vi "Any.vi"(8 "input valid":bool=TRUE, 10 "Value":bool, 11 "Reset":bool) -> (0 "output valid":bool, 2 "Any?":bool)   [LabVIEW 2013]
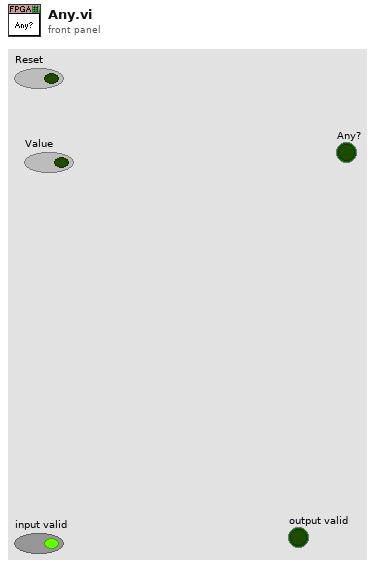
[diagram p1: front panel]
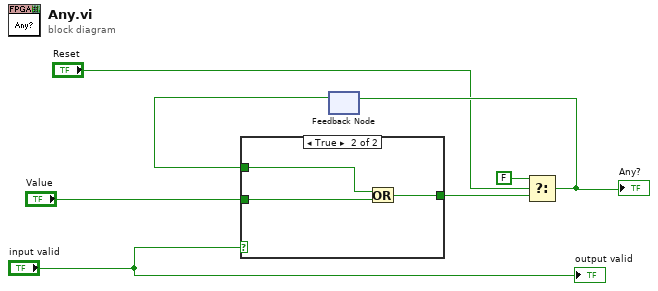
[diagram p0: block diagram]
diagram:
  n1 = feedback #1() -> (w6:bool)  [unwired: 1 in]
  n2 = case shown="True" "input valid" {
    tunnel: "Value" -> [_ w11]
    tunnel: [w8 w10] -> w4
    tunnel: w6 -> [w8 w9]
    frame False {
    }
    frame True {
      n3 = Or(x=w9, y=w11) -> (x .or. y?=w10:bool)
    }
  }
  n4 = Select(t=FALSE, s="Reset", f=w4) -> (s? t:f=w3:bool)
  "Any?" <- w3
  n5 = feedback-in #1(w3) -> ()
  "output valid" <- "input valid"
